vi "Main_008.vi"() -> ()   [LabVIEW 2025]
uses:
  Utility/Universal Utility/TypeDefs_Utility/Cluster_Row-Column.ctl
  9e3f57c0-2ef8-4495-8287-c6a42a5fb955.vi
  Utility/Universal Utility/TypeDefs_Utility/ENUM_4 Directions U-D-L-R.ctl
  Utility/Universal Utility/TypeDefs_Utility/ENUM_8 Directions U-D-L-R.ctl
panel:
  out "Array":u64[][](array[numeric])
  out "number":u64[](array[numeric])
  in  "Number Data":string
  out "MATCH":bool
  in  "Select Data":enum32{"Example", "Puzzle"}(tab)
  in  "EX Target":u64=5832
  in  "Example Input":u64=4
  in  "Puzzle Input":u64=13
  in  "Puzzle Target":u64=23514624000
  out "Answer":u64
  # "TREAT THE DATA AS ONE CONTINUOUS STRING\nNOT AS A 2D ARRAY"
  # "64497254400"
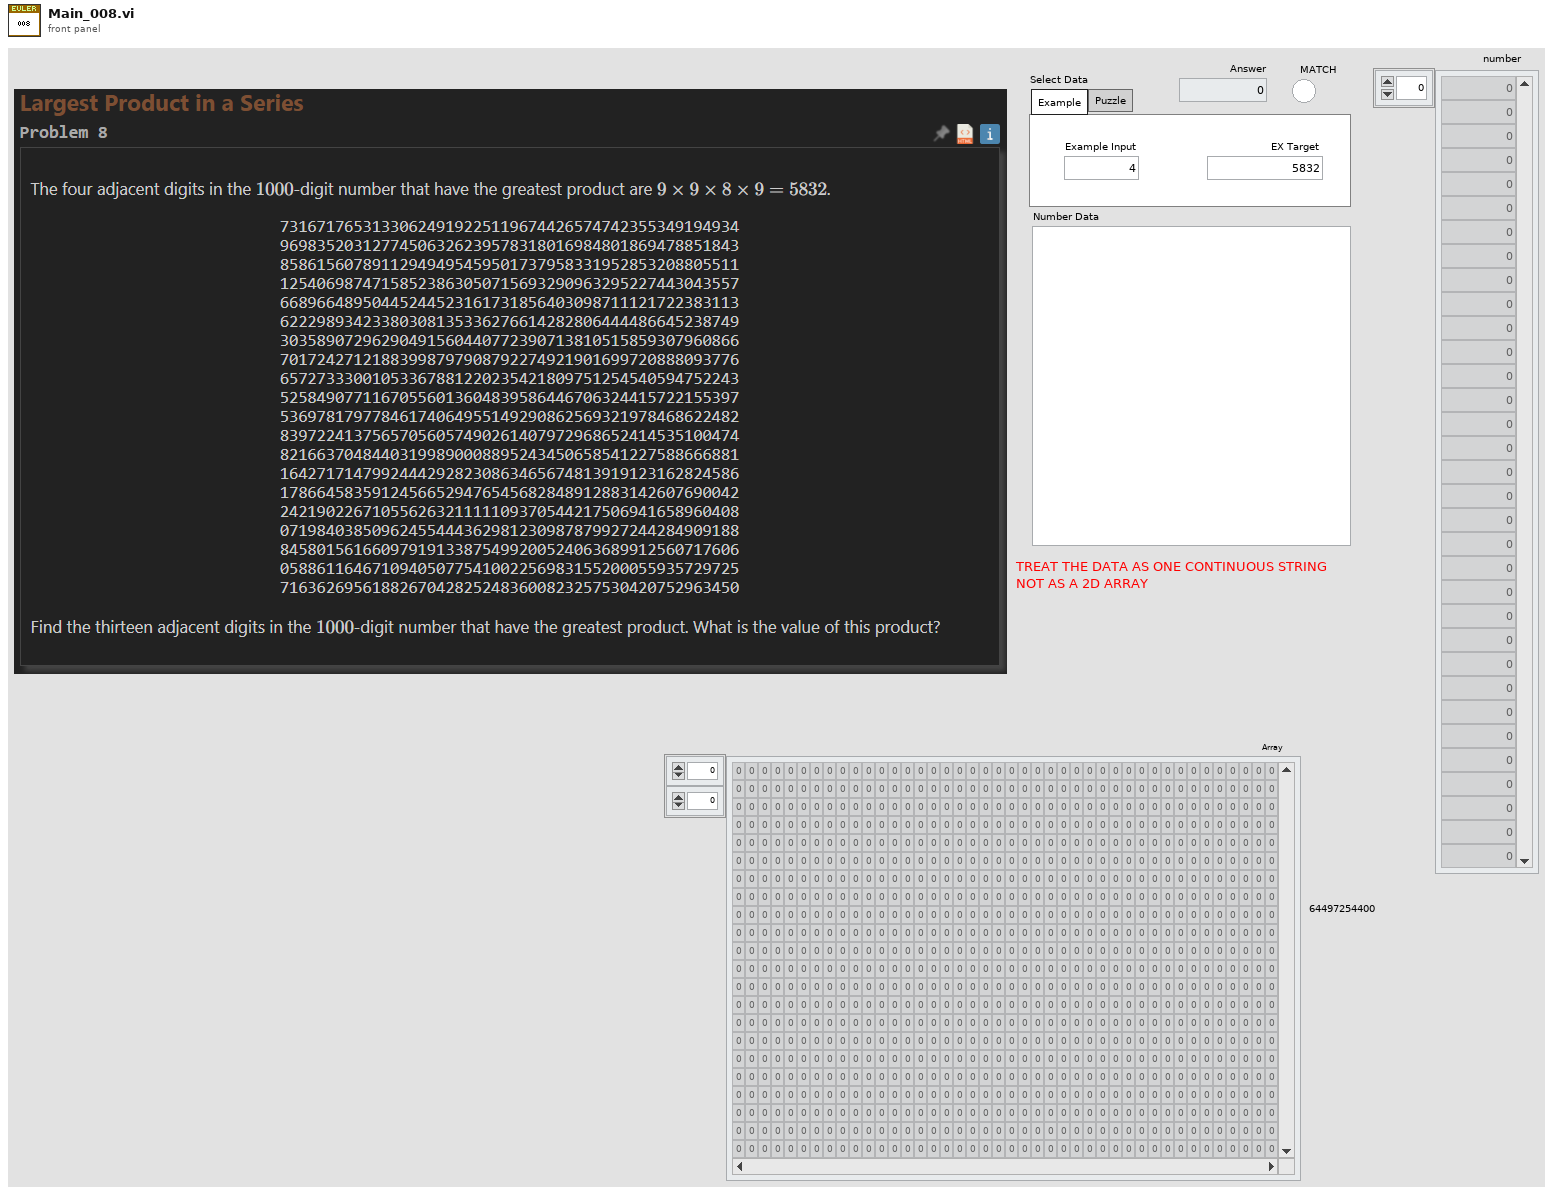
[diagram p1: front panel]
types:
  T1 = typedef "ENUM_8 Directions U-D-L-R.ctl" = enum16{"Up;-1,0", "Up-Right;-1,1", "Right;0,1", "Down-Right;1,1", "Down;1,0", "Down-Left;1,-1", "Left;0,-1", "Up-Left;-1,-1"}
  T2 = typedef "ENUM_4 Directions U-D-L-R.ctl" = enum16{"Up;-1,0", "Right;0,1", "Down;1,0", "Left;0,-1"}
  T3 = typedef "Cluster_Row-Column.ctl" = cluster{"R":i32, "C":i32}
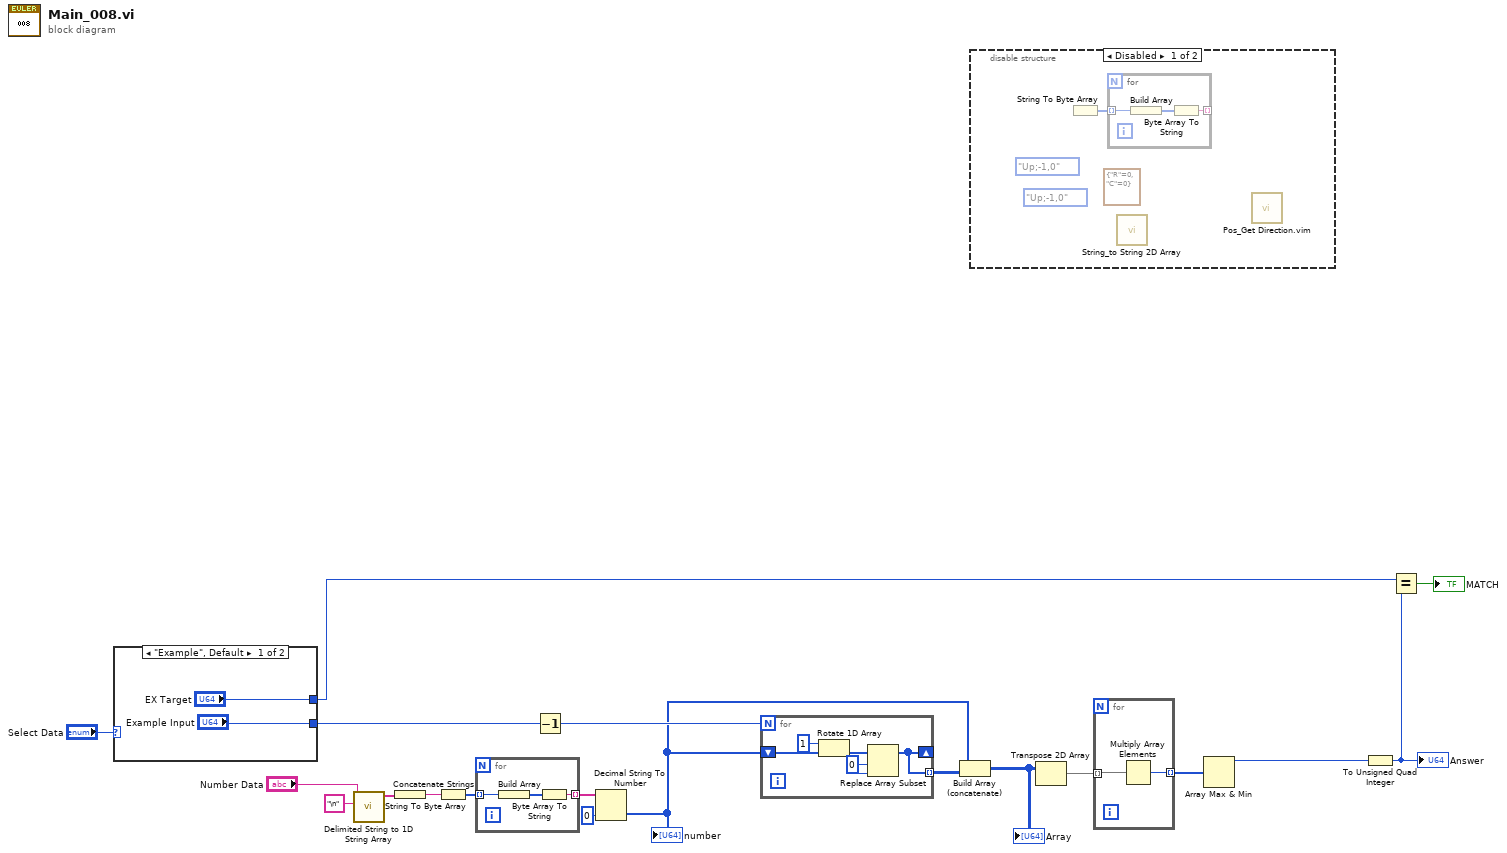
[diagram p0: block diagram]
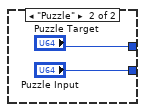
[diagram p2: hidden frame]
diagram:
  n1 = case shown="\"Example\", Default" "Select Data" {
    tunnel: ["Example Input" "Puzzle Input"] -> w13
    tunnel: ["EX Target" "Puzzle Target"] -> w17
    frame "Example", Default {
    }
    frame "Puzzle" {
    }
  }
  n2 = call <vilib>:"Delimited String to 1D String Array.vi"("delimiter"="\n", "delimited string"="Number Data") -> ("string array"=w12:string[])  [unwired: 9 in]
  n3 = Concatenate Strings(w12) -> (w10:string)
  n4 = String To Byte Array(string=w10) -> (unsigned byte array=w11:u8[])
  n5 = for {
    tunnel: w11 -> [w26] mode=indexing
    tunnel: [w24] -> w9 mode=indexing
    n6 = Build Array(w26) -> (w25:u8[])
    n7 = Byte Array To String(unsigned byte array=w25) -> (string=w24:string)
  }
  n8 = Decrement(x=w13) -> (x-1=w7:u64)
  n9 = Decimal String To Number(string=w9, default (0L)=u64 0 ("default (0 I32)")) -> (number=w1:u64[])  [unwired: 1 in, 1 out]
  "number" <- w1
  n10 = for {
    N: w7 -> [_]
    shift-right: [w27] -> _
    shift-left: w1 -> [w31]
    tunnel: [w27] -> w6 mode=indexing
    w29 = u8 0 ("index")
    n11 = Rotate 1D Array(1:w31, 2:1 ("n")) -> (0:w30:u64[])
    n12 = Replace Array Subset(array=w30, new element=w29, index=w29) -> (w27:u64[])
  }
  n13 = Build Array (concatenate)(w1, w6) -> (w2:u64[][])
  "Array" <- w2
  n14 = disable-structure shown="Disabled" {
    frame Disabled {
      (unwired) ENUM_8_Directions_U-D-L-R."Up;-1,0" ("Direction 8")
      (unwired) ENUM_4_Directions_U-D-L-R."Up;-1,0" ("Direction")
      (unwired) T3 {"R"=0, "C"=0} ("Position")
      n15 = String To Byte Array() -> (unsigned byte array=w32:u8[])  [unwired: 1 in]
      n16 = for {
        tunnel: w32 -> [w35] mode=indexing
        tunnel: [w33] -> _ mode=indexing
        n17 = Build Array(w35) -> (w34:u8[])
        n18 = Byte Array To String(unsigned byte array=w34) -> (string=w33:string)
      }
      n19 = call "String_to String 2D Array.vi"() -> ()  [unwired: 11 in, 1 out]
      n20 = call "Pos_Get Direction.vim"() -> ()  [unwired: 11 in, 1 out]
    }
    frame Enabled {
    }
  }
  n21 = Transpose 2D Array(2D array=w2) -> (transposed array=w5:u64[][])
  n22 = for {
    tunnel: w5 -> [w37] mode=indexing
    tunnel: [w36] -> w4 mode=indexing
    n23 = Multiply Array Elements(1:w37) -> (0:w36:u64)
  }
  n24 = Array Max & Min(array=w4) -> (max value=w3:u64)  [unwired: 3 out]
  n25 = To Unsigned Quad Integer(1:w3) -> (0:w16:u64)
  "Answer" <- w16
  n26 = Equal?(x=w17, y=w16) -> (x = y?=→"MATCH":bool)
